vi "Write String to Log.vi"(8 "error in (no error)":errorcluster, 9 "name prefix":string, 11 "file reference in":refnum<file>) -> (0 "error out":errorcluster, 3 "file reference out":refnum<file>)   [LabVIEW 2024]
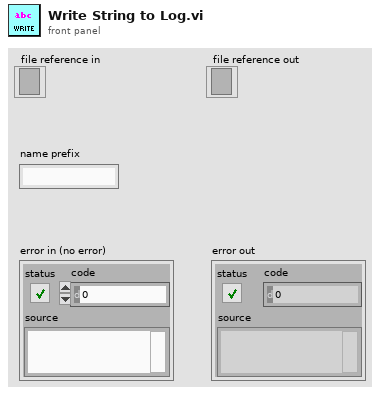
[diagram p1: front panel]
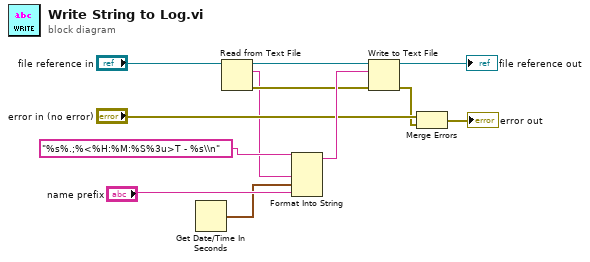
[diagram p0: block diagram]
diagram:
  n1 = Get Date/Time In Seconds() -> (seconds since 1Jan1904=w9:timestamp)
  n2 = Read from Text File(file (use dialog)="file reference in") -> (refnum out=w3:refnum<file>, text=w1:string, error out=w2:errorcluster)  [unwired: 3 in, 1 out]
  n3 = Format Into String(format string="%s%.;%<%H:%M:%S%3u>T - %s\\n" ("Local Time"), w1, w9, "name prefix") -> (resulting string=w8:string)  [unwired: 2 in, 1 out]
  n4 = Write to Text File(file (use dialog)=w3, text=w8, error in=w2) -> (refnum out=→"file reference out":refnum<file>, error out=w6:errorcluster)  [unwired: 1 in, 1 out]
  n5 = Merge Errors("error in (no error)", w6) -> (→"error out":errorcluster)
